vi "String Length in Bytes.vi"(8 "error in (no error)":errorcluster, 11 "UTF8 in":refnum<class "UTF-8 String.lvclass">) -> (0 "error out":errorcluster, 2 "Length in Bytes":i32, 3 "UTF8 out":refnum<class "UTF-8 String.lvclass">)   [LabVIEW 2019, in "JKI Unicode.lvlib" / "UTF-8 String.lvclass"]
doc: "JKI Unicode 1.0.0.7\nTomi Maila - JKI\nCopyright (c) 2016, JKI"
uses:
  UTF-8 String.lvclass
  UTF-8 String.lvclass/UTF-8 String.ctl
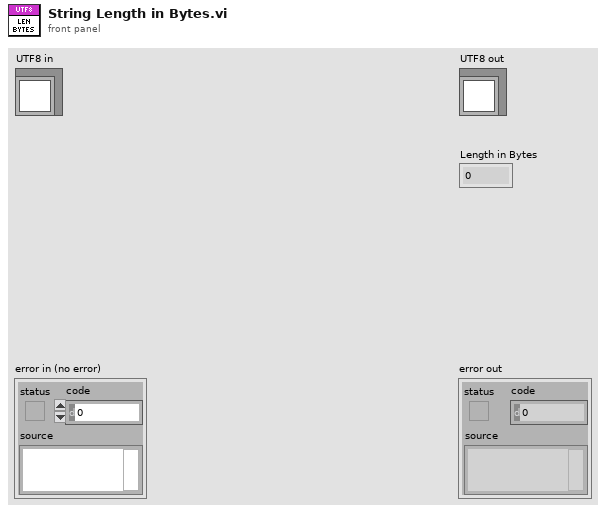
[diagram p1: front panel]
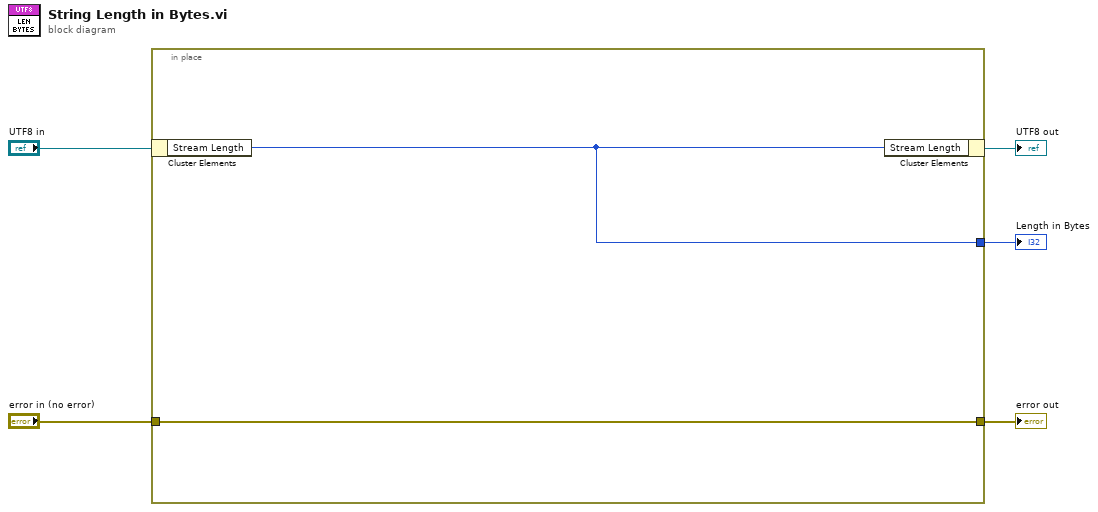
[diagram p0: block diagram]
diagram:
  n1 = in-place {
    in-place-border: "error in (no error)" -> [w6]
    in-place-border: [w7] -> w1
    in-place-border: [w6] -> w4
    n2 = in-place-cluster #1("UTF8 in") -> ("Stream Length"=w7:i32)
    n3 = in-place-cluster #1("Stream Length"=w7) -> (→"UTF8 out":refnum<class "UTF-8 String.lvclass">)
  }
  "error out" <- w4
  "Length in Bytes" <- w1
